vi "ScaledWaveform-AddSection.vi"(8 "Error in":errorcluster, 11 "Custom Device ref":T1 format="%.0x") -> (0 "Error out":errorcluster, 3 "Custom Device ref out":T1 format="%.0x")   [LabVIEW 2015, in "Waveform-Processing-Custom-Device Shared.lvlib" / "Scaled Waveform.lvlib"]
uses:
  Scaled Waveform.lvlib
  <vilib>/NI VeriStand/Custom Device API/Custom Device API.lvlib
  Constants.vi
  Waveform-Processing-Custom-Device Shared.lvlib
  <vilib>/NI Veristand/Custom Device API/Set Item Property (Dependent Node Pointer).vi
  <vilib>/NI Veristand/Custom Device API/Custom Device Item Ref.ctl
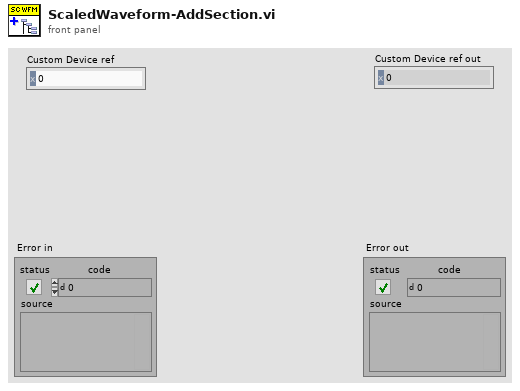
[diagram p1: front panel]
types:
  T1 = typedef "Custom Device API.lvlib/Custom Device Item Ref.ctl" = u64
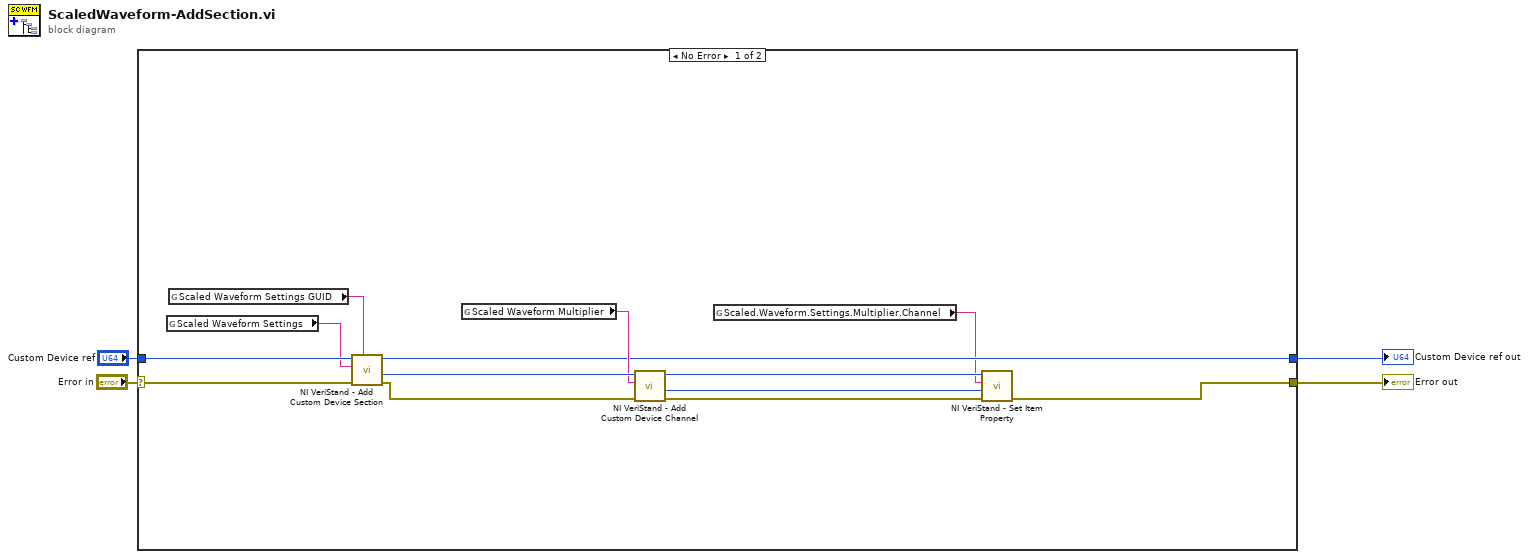
[diagram p0: block diagram]
diagram:
  n1 = case shown="No Error" "Error in" {
    selector: "Error in" -> [w17 w19]
    tunnel: "Custom Device ref" -> [w16 w18]
    tunnel: [w6 w19] -> w2
    tunnel: [w7 w18] -> w1
    frame No Error {
      n2 = global read "Constants.vi" "Scaled Waveform Settings"() -> (w15:string)
      n3 = global read "Constants.vi" "Scaled Waveform Settings GUID"() -> (w14:string)
      n4 = call <vilib>:"NI VeriStand - Add Custom Device Section.vi"("GUID (Default Section)"=w14, "error in (no error)"=w17, "Section Name"=w15, "Parent Ref in"=w16) -> ("error out"=w12:errorcluster, "Section Ptr"=w13:T1, "Parent Ref out"=w7:T1)  [unwired: 4 in, 1 out]
      n5 = global read "Constants.vi" "Scaled Waveform Multiplier"() -> (w11:string)
      n6 = call <vilib>:"NI VeriStand - Add Custom Device Channel.vi"("error in (no error)"=w12, "Channel Name"=w11, "Parent Ref in"=w13) -> ("error out"=w9:errorcluster, "Channel Ref"=w8:T1, "Parent Ref out"=w10:T1)  [unwired: 5 in, 1 out]
      n7 = global read "Constants.vi" "Scaled.Waveform.Settings.Multiplier.Channel"() -> (w5:string)
      n8 = call-poly <vilib>:"NI VeriStand - Set Item Property.vi"("error in (no error)"=w9, "Dependent Node Ref"=w8, "Property Name"=w5, "Item Ref in"=w10) -> ("error out"=w6:errorcluster)  [unwired: 5 in, 2 out]
    }
    frame Error {
    }
  }
  "Error out" <- w2
  "Custom Device ref out" <- w1
